vi "Arduino_wait_for_signal_serial.vi"(8 "error in (no error)":errorcluster, 10 "time to wait/s":i32, 11 "reference":refnum<visa-resource-name>) -> (0 "error out":errorcluster, 2 "String":string="No signal detected", 3 "VISA resource name out":refnum<visa-resource-name>)   [LabVIEW 2015]
panel:
  out "String 2":string
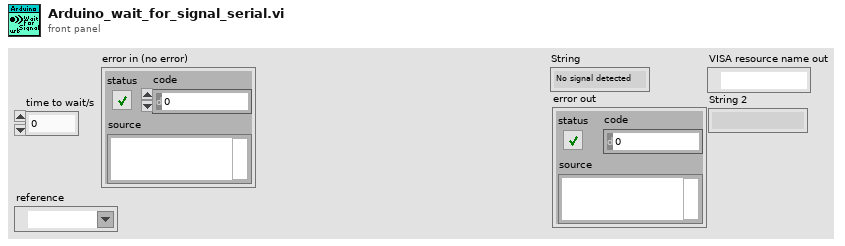
[diagram p1: front panel]
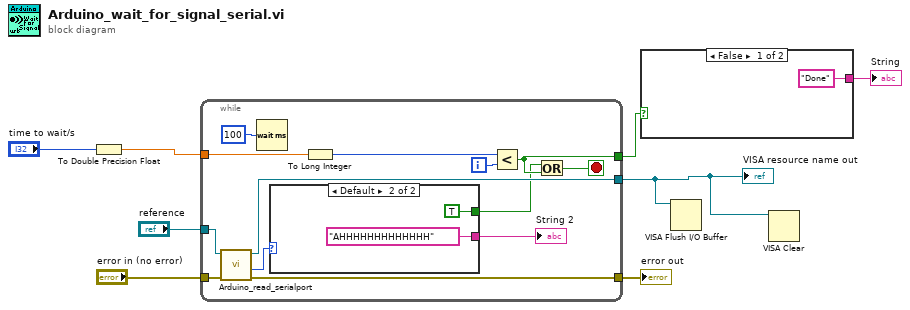
[diagram p0: block diagram]
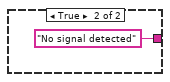
[diagram p2: hidden frame]
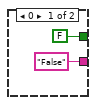
[diagram p3: hidden frame]
diagram:
  n1 = To Double Precision Float(number="time to wait/s") -> (double precision float=w2:dbl)
  n2 = while {
    tunnel: w2 -> [w18]
    tunnel: "error in (no error)" -> [w14]
    tunnel: [w16] -> w6
    tunnel: "reference" -> [w15]
    tunnel: [w13] -> w1
    tunnel: [w12] -> w3
    i -> [w20]
    stop <- w19 stop-if-true
    n3 = call "Arduino_read_serialport.vi"("error in (no error)"=w14, "reference"=w15) -> ("error out"=w12:errorcluster, "Bytes at Port"=w9:u32, "VISA resource name out"=w13:refnum<visa-resource-name>)  [unwired: 6 in, 1 out]
    n4 = Wait (ms)(milliseconds to wait=u32 100) -> ()  [unwired: 1 out]
    n5 = case shown="Default" w9 {
      tunnel: [FALSE TRUE] -> w11
      tunnel: ["False" "AHHHHHHHHHHHHH"] -> w10
      frame 0 {
      }
      frame Default {
      }
    }
    "String 2" <- w10
    n6 = To Long Integer(number=w18) -> (32bit integer=w17:i32)
    n7 = Less?(x=w17, y=w20) -> (x < y?=w16:bool)
    n8 = Or(x=w11, y=w16) -> (x .or. y?=w19:bool)
  }
  "error out" <- w3
  "VISA resource name out" <- w1
  n9 = case shown="False" w6 {
    tunnel: ["Done" "No signal detected"] -> w5
    frame False {
    }
    frame True {
    }
  }
  "String" <- w5
  n10 = VISA Flush I/O Buffer(VISA resource name=w1) -> ()  [unwired: 2 in, 2 out]
  n11 = VISA Clear(VISA resource name=w1) -> ()  [unwired: 1 in, 2 out]
